vi "Get Classes Names.vi"() -> (3 "Array":string[](array[string]))   [LabVIEW 2020, in "Oscilloscope.lvlib"]
uses:
  Oscilloscope.lvlib
  Clases/Osciloscopio/Osciloscopio.lvclass
  Clases/TDS 2000/TDS 2000.lvclass
  C:/Users/ronad/Osciloscopio/Osciloscopio DQMH/Libraries/Oscilloscope/Clases/Osciloscopio/Osciloscopio.lvclass
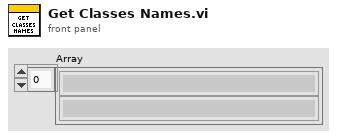
[diagram p1: front panel]
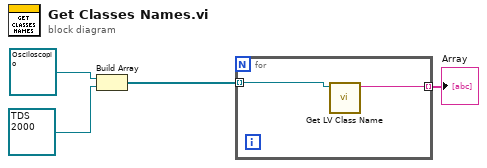
[diagram p0: block diagram]
diagram:
  n1 = Build Array(refnum<class "Osciloscopio.lvclass"> refnum ("Oscilloscope.lvlib:Osciloscopio.lvclass"), refnum<class "TDS 2000.lvclass"> refnum ("Oscilloscope.lvlib:TDS 2000.lvclass")) -> (w2:refnum<class "Osciloscopio.lvclass">[])
  n2 = for {
    tunnel: w2 -> [w6] mode=indexing
    tunnel: [w5] -> w1 mode=indexing
    n3 = call <vilib>:"Get LV Class Name.vi"("object"=w6) -> ("class name"=w5:string)  [unwired: 9 in, 1 out]
  }
  "Array" <- w1
